vi "dosimat_init.vi"(3 "Dosimat Port In":refnum<visa-resource-name>="COM1") -> (0 "error out":errorcluster, 1 "Dosimat Port Out":refnum<visa-resource-name>="COM1")   [LabVIEW 2010]
uses:
  <vilib>/Instr/_visa.llb/VISA Configure Serial Port (Instr).vi
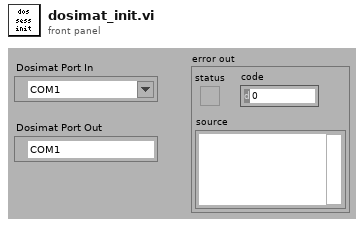
[diagram p1: front panel]
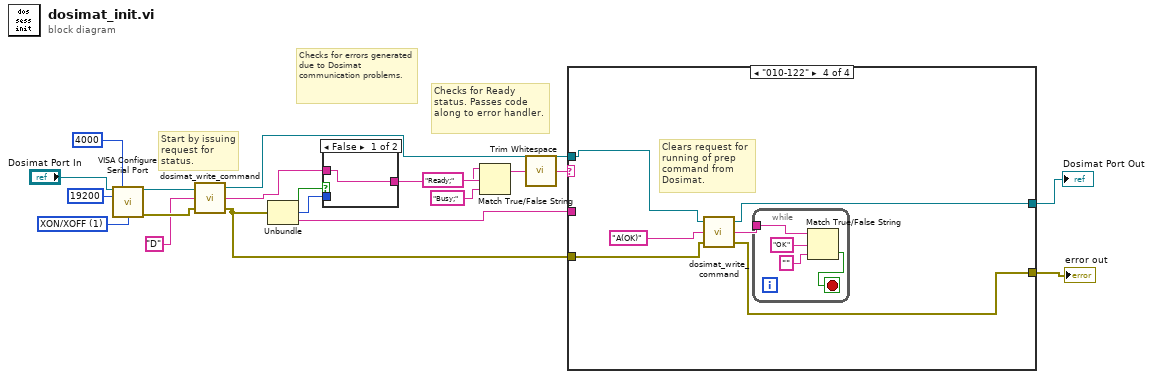
[diagram p0: block diagram]
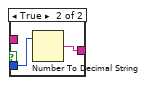
[diagram p2: hidden frame]
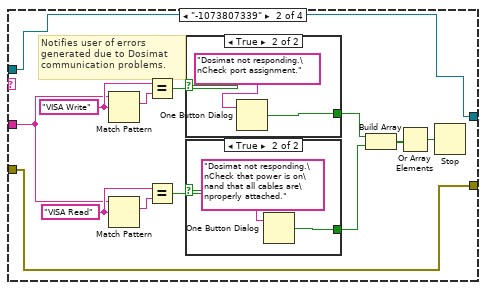
[diagram p4: hidden frame]
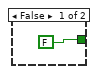
[diagram p5: hidden frame]
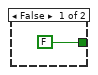
[diagram p6: hidden frame]
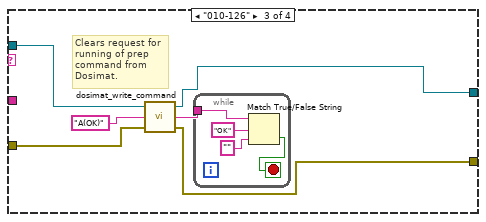
[diagram p7: hidden frame]
diagram:
  w18 = u16 1 items=["None", "XON/XOFF", "RTS/CTS", "XON/XOFF & RTS/CTS", "DTR/DSR", "XON/XOFF & DTR/DSR"] ("flow control (0:none)")
  # "Checks for Ready status. Passes code along to error handler."
  # "Start by issuing request for status."
  # "Checks for errors generated due to Dosimat communication problems."
  n1 = call-poly "VISA Configure Serial Port"("VISA resource name"="Dosimat Port In", "timeout (10sec)"=u32 4000, "baud rate (9600)"=u32 19200, "flow control (0:none)"=w18) -> ("VISA resource name out"=w7:refnum<visa-resource-name>, "error out"=w6:errorcluster)  [unwired: 10 in]
  n2 = call "dosimat_write_command.vi"("error in"=w6, "write buffer"="D", "Dosimat Port In"=w7) -> ("error out"=w4:errorcluster, "read buffer"=w13:string, "Dosimat Port Out"=w2:refnum<visa-resource-name>)
  n3 = Unbundle(w4) -> ("status"=w14:bool, "code"=w15:i32, "source"=w16:string)
  n4 = case shown="False" w14 {
    tunnel: w15 -> [_ w23]
    tunnel: [w21 w22] -> w9
    tunnel: w13 -> [w21 _]
    frame False {
    }
    frame True {
      n5 = Number To Decimal String(number=w23) -> (decimal integer string=w22:string)  [unwired: 1 in]
    }
  }
  n6 = Match True/False String(2:"Busy;" ("false string"), 3:"Ready;" ("true string"), 4:w9) -> (1:w10:string)  [unwired: 1 out]
  n7 = call <vilib>:"Trim Whitespace.vi"("string"=w10) -> ("trimmed string"=w8:string)  [unwired: 1 in]
  n8 = case shown="\"010-122\"" w8 {
    tunnel: w16 -> [_ w32 _ _]
    tunnel: w4 -> [w24 w26 w48 w58]
    tunnel: [w24 w26 w49 w57] -> w3
    tunnel: w2 -> [w25 w27 w46 w56]
    tunnel: [w25 w27 w45 w55] -> w1
    frame "0", Default {
      # "No error detected yet."
    }
    frame "-1073807339" {
      w34 = "VISA Read" ("regular expression")
      w37 = "VISA Write" ("regular expression")
      # "Notifies user of errors generated due to Dosimat communication problems."
      n9 = Match Pattern(string=w32, regular expression=w37) -> (match substring=w38:string)  [unwired: 1 in, 3 out]
      n10 = Match Pattern(string=w32, regular expression=w34) -> (match substring=w33:string)  [unwired: 1 in, 3 out]
      n11 = Equal?(x=w37, y=w38) -> (x = y?=w36:bool)
      n12 = Equal?(x=w34, y=w33) -> (x = y?=w35:bool)
      n13 = case shown="True" w36 {
        tunnel: [FALSE w43] -> w29
        frame False {
        }
        frame True {
          n14 = One Button Dialog(message="Dosimat not responding.\nCheck port assignment.") -> (true=w43:bool)  [unwired: 1 in]
        }
      }
      n15 = case shown="True" w35 {
        tunnel: [FALSE w40] -> w30
        frame False {
        }
        frame True {
          n16 = One Button Dialog(message="Dosimat not responding.\nCheck that power is on\nand that all cables are\nproperly attached.") -> (true=w40:bool)  [unwired: 1 in]
        }
      }
      n17 = Build Array(w29, w30) -> (w28:bool[])
      n18 = Or Array Elements(Boolean array=w28) -> (logical OR=w31:bool)
      n19 = Stop(stop? (T)=w31) -> ()
    }
    frame "010-126" {
      # "Clears request for running of prep command from Dosimat."
      n20 = call "dosimat_write_command.vi"("error in"=w48, "write buffer"="A(OK)", "Dosimat Port In"=w46) -> ("error out"=w49:errorcluster, "read buffer"=w50:string, "Dosimat Port Out"=w45:refnum<visa-resource-name>)
      n21 = while {
        tunnel: w50 -> [w51]
        stop <- w52 stop-if-true
        n22 = Match True/False String(2:"" ("false string"), 3:"OK" ("true string"), 4:w51) -> (0:w52:bool)  [unwired: 1 out]
      }
    }
    frame "010-122" {
      # "Clears request for running of prep command from Dosimat."
      n23 = call "dosimat_write_command.vi"("error in"=w58, "write buffer"="A(OK)", "Dosimat Port In"=w56) -> ("error out"=w57:errorcluster, "read buffer"=w59:string, "Dosimat Port Out"=w55:refnum<visa-resource-name>)
      n24 = while {
        tunnel: w59 -> [w61]
        stop <- w62 stop-if-true
        n25 = Match True/False String(2:"" ("false string"), 3:"OK" ("true string"), 4:w61) -> (0:w62:bool)  [unwired: 1 out]
      }
    }
  }
  "error out" <- w3
  "Dosimat Port Out" <- w1
